vi "Insert Module Types.vi"(10 "All Modules types":T1[](array[typedef]), 11 "Project info Results In":string[][](array[string])) -> (3 "Project info Results Out":string[][](array[string]))   [LabVIEW 2019, in "Panther Dashboard.lvlib"]
uses:
  Panther Dashboard.lvlib
  Module type--enum.ctl
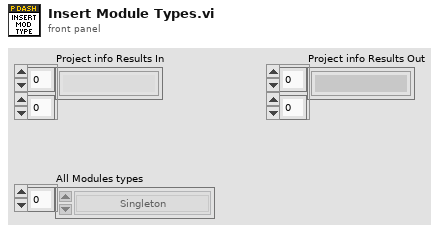
[diagram p1: front panel]
types:
  T1 = typedef "Panther Dashboard.lvlib/Module type--enum.ctl" = enum16{"Singleton", "Cloneable"}
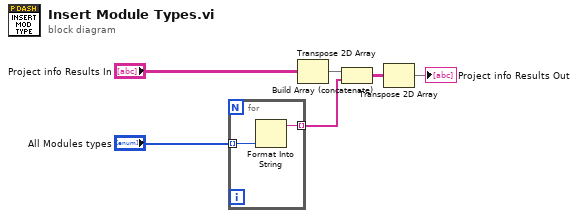
[diagram p0: block diagram]
diagram:
  n1 = for {
    tunnel: "All Modules types" -> [w8] mode=indexing
    tunnel: [w7] -> w5 mode=indexing
    n2 = Format Into String(w8) -> (resulting string=w7:string)  [unwired: 3 in, 1 out]
  }
  n3 = Transpose 2D Array(2D array="Project info Results In") -> (transposed array=w2:string[][])
  n4 = Build Array (concatenate)(w2, w5) -> (w6:string[][])
  n5 = Transpose 2D Array(2D array=w6) -> (transposed array=→"Project info Results Out":string[][])
